vi "Nested Loops 1234,1234.vi"() -> ()   [LabVIEW 2019]
panel:
  out "Counter":dbl(slide) scale=1.0..4.0
  in  "Push button to stop program":bool
  # "Challenge:\n1234,1234. Write a program that counts to four repeatedly."
  # "Try it: Run the program and watch the counter."
  # "You will probably need:\nNested loops, for loop, while loop, indicators, wait for ms, numeric functions"
  # "Open the block diagram to see a possible solution."
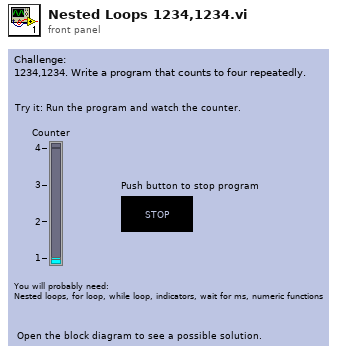
[diagram p1: front panel]
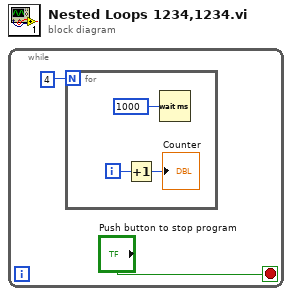
[diagram p0: block diagram]
diagram:
  n1 = while {
    stop <- "Push button to stop program" stop-if-true
    n2 = for {
      N: 4 -> [_]
      i -> [w4]
      n3 = Increment(x=w4) -> (x+1=→"Counter":i32)
      n4 = Wait (ms)(milliseconds to wait=1000) -> ()  [unwired: 1 out]
    }
  }
